vi "Set Acceleration Feed-Forward Gain.vi"(4 "error in (no error)":errorcluster, 5 "Acceleration feed-forward gain factor (0)":dbl min=0.0 max=2000000000.0 format="%.6g", 6 "Axis (1)":i32=1 min=1 max=3, 7 "VISA resource name":refnum<visa-resource-name>) -> (0 "error out":errorcluster, 3 "VISA resource name out":refnum<visa-resource-name>)   [LabVIEW 2014, in "Newport ESP301.lvlib"]
doc: "This command sets the acceleration feed-forward gain factor Af. It is active for any DC servo based motion device.\n\nSee the \"Feed-Forward Loops\" in Motion Control Tutorial section (ESP301 User's manual.pdf) to understand the basic principles of feed-forward.\n\n<B>Note:</B> The command can be sent at any time but it has no effect until the UF (update filter) is received."
uses:
  Newport ESP301.lvlib
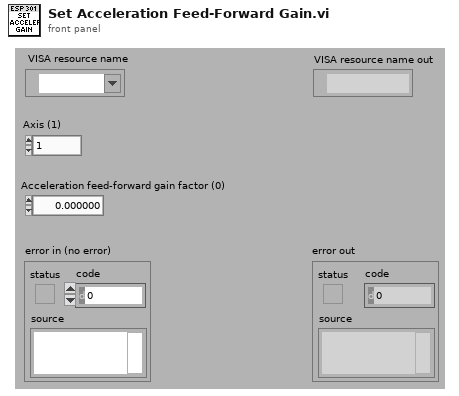
[diagram p1: front panel]
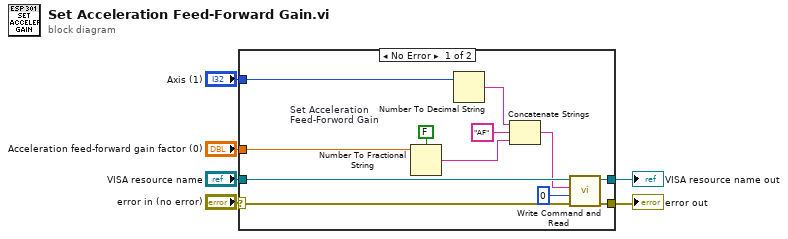
[diagram p0: block diagram]
diagram:
  n1 = case shown="No Error" "error in (no error)" {
    selector: "error in (no error)" -> [w9 w20]
    tunnel: [w7 w20] -> w6
    tunnel: "VISA resource name" -> [w12 w19]
    tunnel: [w8 w19] -> w5
    tunnel: "Axis (1)" -> [w16 _]
    tunnel: "Acceleration feed-forward gain factor (0)" -> [w15 _]
    frame No Error {
      w18 = "AF"  # Set Acceleration Feed-Forword Gain
      n2 = Number To Fractional String(use system decimal point (T)=FALSE ("utiliser le séparateur décimal du système (V)"), number=w15) -> (F-format string=w14:string)  [unwired: 2 out]
      n3 = Number To Decimal String(number=w16) -> (decimal integer string=w17:string)  [unwired: 1 out]
      n4 = Concatenate Strings(w17, w18, w14) -> (w11:string)
      n5 = call "Write Command and Read.vi"("error in (no error)"=w9, "Bytes to read (100)"=u32 0, "Command"=w11, "VISA resource name"=w12) -> ("error out"=w7:errorcluster, "VISA resource name out"=w8:refnum<visa-resource-name>)  [unwired: 1 in, 3 out]
    }
    frame Error {
    }
  }
  "error out" <- w6
  "VISA resource name out" <- w5
